vi "Validate Payload.vi"(8 "error in (no error)":errorcluster, 11 "ControlPacket in":refnum<class "ControlPacket.lvclass">) -> (0 "error out":errorcluster, 1 "valid?":bool, 3 "ControlPacket out":refnum<class "ControlPacket.lvclass">)   [LabVIEW 2013, in "MQTT_Control_Packets.lvlib" / "ControlPacket.lvclass"]
uses:
  ControlPacket.lvclass
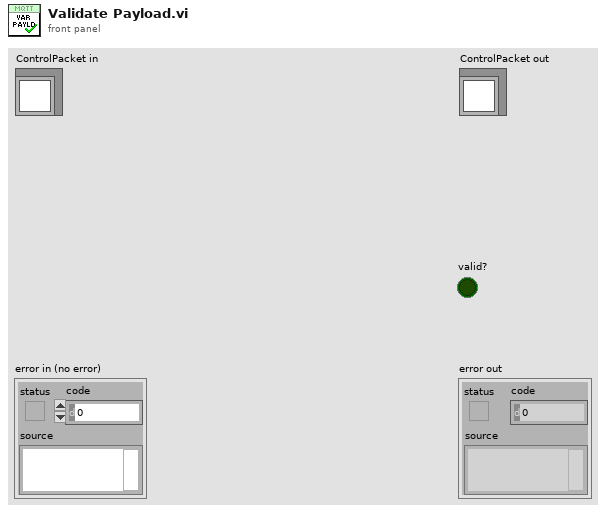
[diagram p1: front panel]
types:
  T1 = typedef "MQTT_Control_Packets.lvlib/ControlPacket.lvclass/Requirement -- enum.ctl" = enum16{"None", "Optional", "Required"}
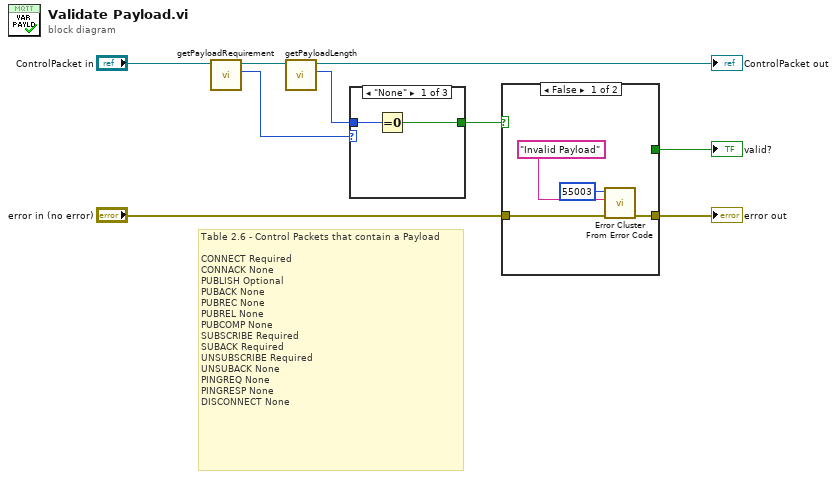
[diagram p0: block diagram]
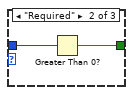
[diagram p2: hidden frame]
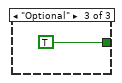
[diagram p3: hidden frame]
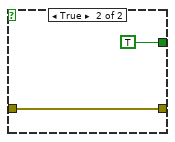
[diagram p4: hidden frame]
diagram:
  # "Table 2.6 - Control Packets that contain a Payload\n\nCONNECT Required\nCONNACK None\nPUBLISH Optional\nPUBACK None\nPUBREC None\nPUBREL None\nPUBCOMP None\nSUBSCRIBE Required\nSUBACK Required\nUNSUBSCRIBE Required\nUNSUBACK None\nPINGREQ None\nPINGRESP None\nDISCONNECT None"
  n1 = call-dynamic "getPayloadRequirement.vi"("ControlPacket in"="ControlPacket in") -> ("Requirement"=w4:T1, "ControlPacket out"=w9:refnum<class "ControlPacket.lvclass">)  [unwired: 9 in]
  n2 = call "getPayloadLength.vi"("ControlPacket in"=w9) -> ("Payload size"=w3:u32, "ControlPacket out"=→"ControlPacket out":refnum<class "ControlPacket.lvclass">)  [unwired: 9 in]
  n3 = case shown="\"None\"" w4 {
    tunnel: w3 -> [w11 w13 _]
    tunnel: [w10 w12 TRUE] -> w2
    frame "None" {
      n4 = Equal To 0?(x=w11) -> (x = 0?=w10:bool)
    }
    frame "Required" {
      n5 = Greater Than 0?(x=w13) -> (x > 0?=w12:bool)
    }
    frame "Optional" {
    }
  }
  n6 = case shown="False" w2 {
    tunnel: [w18 w20] -> w6
    tunnel: "error in (no error)" -> [w15 w20]
    tunnel: [_ TRUE ("valid?")] -> w1
    frame False {
      n7 = call <vilib>:"Error Cluster From Error Code.vi"("error in (no error)"=w15, "error message (\"\")"="Invalid Payload" ("error message (\"\")"), "error code (0)"=55003) -> ("error out"=w18:errorcluster)  [unwired: 6 in]
    }
    frame True {
    }
  }
  "error out" <- w6
  "valid?" <- w1
